vi "Information.vi"(8 "error in":errorcluster, 11 "ref in":refnum<k7>) -> (0 "error out":errorcluster, 1 "height":i32, 2 "width":i32, 3 "ref out":refnum<k7>, 5 "fps":dbl)   [LabVIEW 2010]
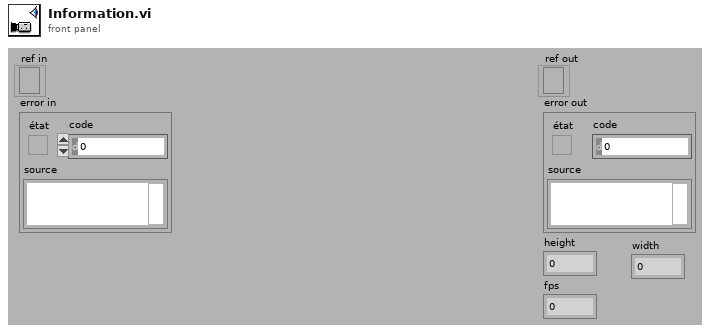
[diagram p1: front panel]
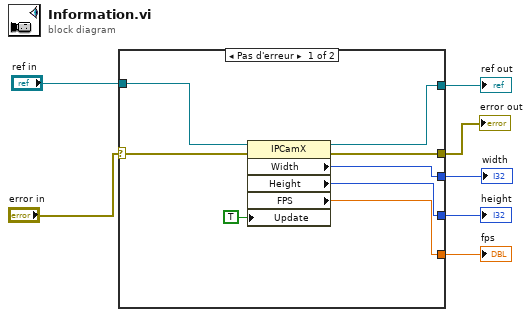
[diagram p0: block diagram]
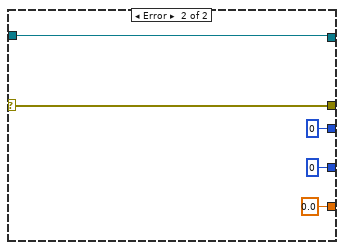
[diagram p2: hidden frame]
diagram:
  n1 = case shown="Pas d'erreur" "error in" {
    selector: "error in" -> [w8 w17]
    tunnel: "ref in" -> [w15 w16]
    tunnel: [w14 w16] -> w6
    tunnel: [w13 w17] -> w5
    tunnel: [w12 0 ("Width")] -> w4
    tunnel: [w11 0 ("Height")] -> w3
    tunnel: [w10 0.0 ("FPS")] -> w2
    frame No Error {
      n2 = property class="IPCamX"(reference=w15, error in=w8, "Update"=TRUE) -> (reference out=w14:refnum<k7>, error out=w13:errorcluster, "Width"=w12:i32, "Height"=w11:i32, "FPS"=w10:dbl)
    }
    frame Error {
    }
  }
  "ref out" <- w6
  "error out" <- w5
  "width" <- w4
  "height" <- w3
  "fps" <- w2
